vi "KPRO State Controller 2016.vi"(0 "Start KPRO":bool, 1 "Start Slug Test":bool, 2 "Start YSI Capture":bool, 3 "Clear Volume":bool, 4 "Capture Head Pressure":bool, 5 "Done":bool, 6 "Previous \nState":i32, 7 "Change Settings":bool) -> (11 "State String":string, 12 "Next State":i32, 13 "State Changed":bool, 14 "Start KPRO Enabler":u8, 15 "Start Slug Test Enabler":u8, 16 "Start YSI Capture Enabler":u8, 17 "Clear Volume Enabler":u8, 18 "Capture Head Pressure Enabler":u8, 19 "Change Settings Enabler":u8)   [LabVIEW 2016]
doc: "This VI takes in the Button State, Previous State and the Done Input and Generates the Next State, the string which indicates the current state, indicates if a state change has occurred and sets the enable/disable line on the buttons to guide the user through the possible states."
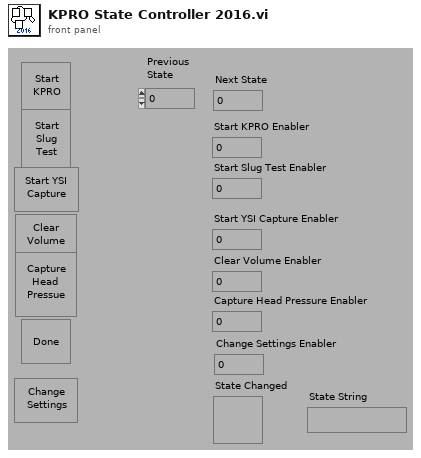
[diagram p1: front panel]
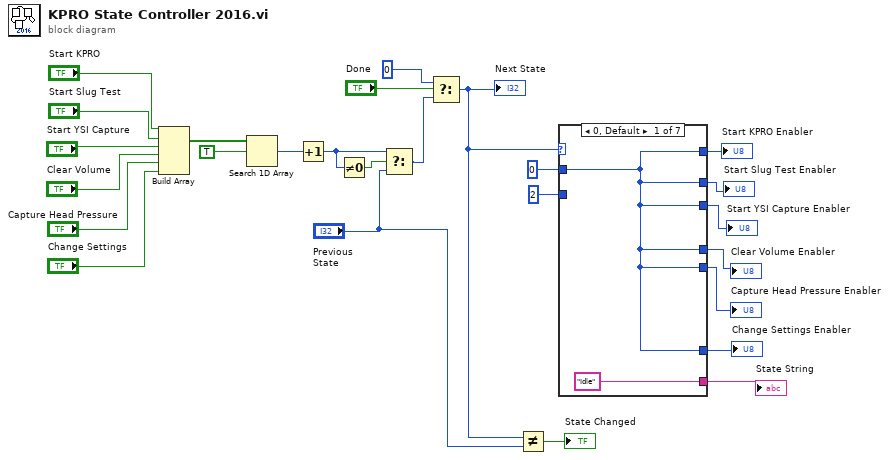
[diagram p0: block diagram]
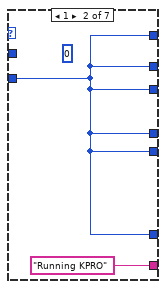
[diagram p2: hidden frame]
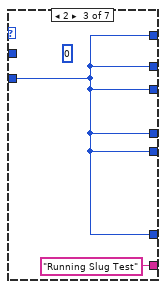
[diagram p3: hidden frame]
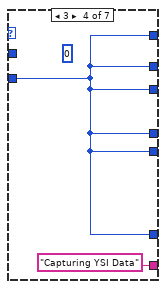
[diagram p4: hidden frame]
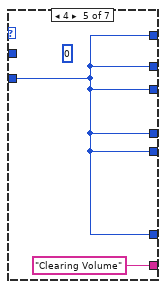
[diagram p5: hidden frame]
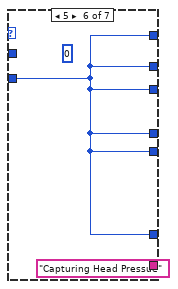
[diagram p6: hidden frame]
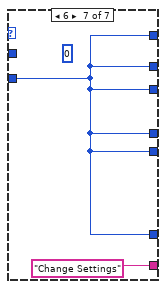
[diagram p7: hidden frame]
diagram:
  n1 = Build Array("Start KPRO", "Start Slug Test", "Start YSI Capture", "Clear Volume", "Capture Head Pressure", "Change Settings") -> (w22:bool[])
  n2 = Search 1D Array(1D array=w22, element=TRUE) -> (index of element=w20:i32)  [unwired: 1 in]
  n3 = Increment(x=w20) -> (x+1=w15:i32)
  n4 = Not Equal To 0?(x=w15) -> (x != 0?=w16:bool)
  n5 = Select(t=w15, s=w16, f="Previous \nState") -> (s? t:f=w17:i32)
  n6 = Select(t=0, s="Done", f=w17) -> (s? t:f=w10:i32)
  "Next State" <- w10
  n7 = Not Equal?(x=w10, y="Previous \nState") -> (x != y?=→"State Changed":bool)
  n8 = case shown="0, Default" w10 {
    tunnel: [w27 w29 w31 w33 w35 w37 w39] -> w13
    tunnel: [w27 w29 w31 w33 w35 w37 w39] -> w12
    tunnel: [w27 w29 w31 w33 w35 w37 w39] -> w11
    tunnel: [w27 w29 w31 w33 w35 w37 w39] -> w7
    tunnel: [w27 w29 w31 w33 w35 w37 w39] -> w6
    tunnel: ["Idle" "Running KPRO" "Running Slug Test" "Capturing YSI Data" "Clearing Volume" "Capturing Head Pressue" "Change Settings"] -> w5
    tunnel: [w27 w29 w31 w33 w35 w37 w39] -> w3
    tunnel: 0 -> [w27 _ _ _ _ _ _]
    tunnel: 2 -> [_ w29 w31 w33 w35 w37 w39]
    frame 0, Default {
    }
    frame 1 {
      (unwired) 0
    }
    frame 2 {
      (unwired) 0
    }
    frame 3 {
      (unwired) 0
    }
    frame 4 {
      (unwired) 0
    }
    frame 5 {
      (unwired) 0
    }
    frame 6 {
      (unwired) 0
    }
  }
  "Start KPRO Enabler" <- w13
  "Start Slug Test Enabler" <- w12
  "Start YSI Capture Enabler" <- w11
  "Clear Volume Enabler" <- w7
  "Capture Head Pressure Enabler" <- w6
  "State String" <- w5
  "Change Settings Enabler" <- w3
